vi "pi.run.vi"(4 "reset? (F)":bool, 5 "discretization_method (trapezoidal)":T1, 6 "output_limits (100/0)":cluster{"max_limit":dbl, "min_limit":dbl}={"max_limit"=100.0, "min_limit"=0.0}, 7 "pi_parameters":cluster{"Kc":dbl, "Ti":dbl}, 8 "sampling_time (s)":dbl, 9 "initial_output (0)":dbl format="%#_13g", 10 "feedback":dbl format="%#_13g", 11 "setpoint":dbl format="%#_13g") -> (3 "controller_output":dbl)   [LabVIEW 2015, in "discrete_control_systems.lvlib"]
doc: "Implements a PI controller in Standard Form using the provided Kc and Ti paramenters and sampling time. \n\nThe implemented controller has the following equation in the LaPlace domain, where U(s) is the controller output:\n\nU(s) = Kc * ( 1 + 1/(Ti*s) )\n\nThe sampling_time input represents how fast will the control loop run and is necessary in order to allow for an accurate implementation of the controller with parameters that can be reused for multiple sampling times.\n\nThe discretization_method can be selected if desired and defaults to trapezoidal. Most users won't need to modify this.\n\nThe reset? input can be used to reinitialize the internal registers for the controller and start from zero.\n\nThe output will be coerced withing min_limit and max_limit. After resetting the controller, the output will be initialized to the initial output selected. This helps implement bumpless transfers between open loop and closed loop operations."
uses:
  discrete_control_systems.lvlib
  typedefs/discretization_method -- enum.ctl
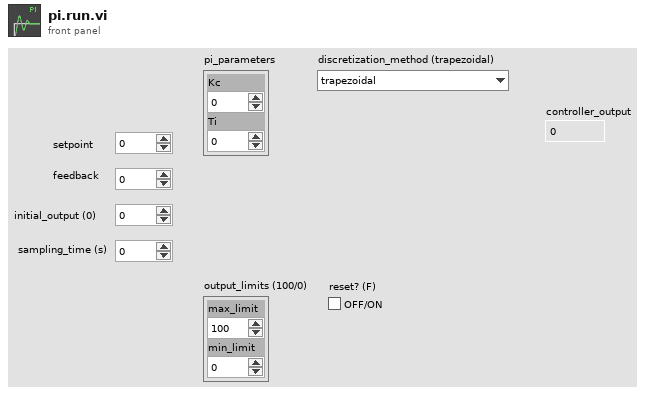
[diagram p1: front panel]
types:
  T1 = typedef "discrete_control_systems.lvlib/discretization_method -- enum.ctl" = enum16{"trapezoidal", "backward_euler"}
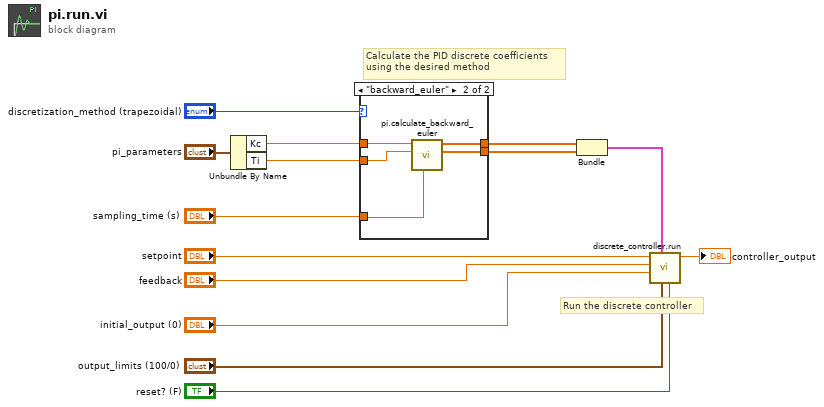
[diagram p0: block diagram]
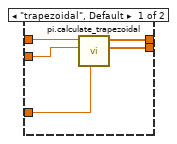
[diagram p2: hidden frame]
diagram:
  # "Run the discrete controller"
  # "Calculate the PID discrete coefficients\nusing the desired method"
  n1 = Unbundle By Name("pi_parameters") -> ("Kc"=w2:dbl, "Ti"=w1:dbl)
  n2 = case shown="\"backward_euler\"" "discretization_method (trapezoidal)" {
    tunnel: w2 -> [w19 w24]
    tunnel: w1 -> [w18 w23]
    tunnel: "sampling_time (s)" -> [w17 w22]
    tunnel: [w16 w21] -> w9
    tunnel: [w15 w20] -> w8
    frame "trapezoidal", Default {
      n3 = call "pi.calculate_trapezoidal.vi"("sampling_time (s)"=w17, "Ti"=w18, "Kc"=w19) -> ("a1...an"=w15:dbl[], "b0...bn"=w16:dbl[])  [unwired: 7 in]
    }
    frame "backward_euler" {
      n4 = call "pi.calculate_backward_euler.vi"("sampling_time (s)"=w22, "Ti"=w23, "Kc"=w24) -> ("a1...an"=w20:dbl[], "b0...bn"=w21:dbl[])  [unwired: 7 in]
    }
  }
  n5 = Bundle("b0...bn"=w9, "a1...an"=w8) -> (w7:cluster{"b0...bn":dbl[], "a1...an":dbl[]})  [unwired: 1 in]
  n6 = call "discrete_controller.run.vi"("reset? (F)"="reset? (F)", "outut limits (100/0)"="output_limits (100/0)", "discrete_coefficients"=w7, "initial_output (0)"="initial_output (0)", "feedback"="feedback", "setpoint"="setpoint") -> ("controller_output"=→"controller_output":dbl)  [unwired: 5 in]
